vi "File Title Dialog.vi"() -> (1 "Accepted":bool, 2 "Additional Description out":string, 3 "File Title out":string="datafile_arduino")   [LabVIEW 2019]
panel:
  in  "Accept":bool
  in  "Additional Description":string
  in  "File Title":string="datafile_arduino"
  # "(no need to specify file extensions)"
  # "Numbers will be added if required to make the main filename unique."
  # "This will be written into the datafiles in the header, and can be left blank if desired. Commas are removed."
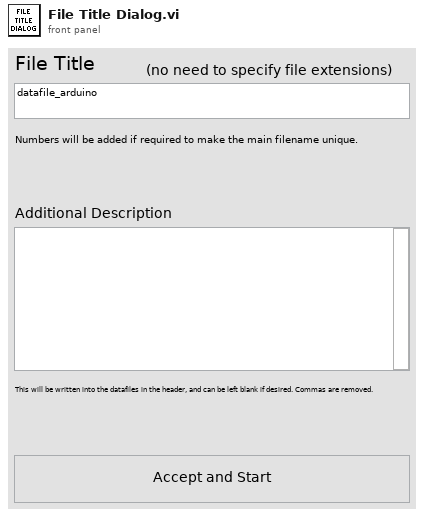
[diagram p1: front panel]
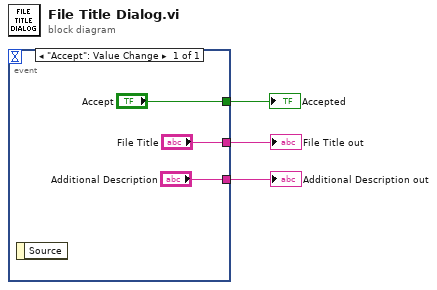
[diagram p0: block diagram]
diagram:
  n1 = event shown="[0] \"Accept\": Value Change" {
    selector: _ -> [_]
    dyn-events: _ -> [_]
    timeout: _ -> [_]
    tunnel: ["Accept"] -> w3
    tunnel: ["File Title"] -> w2
    tunnel: ["Additional Description"] -> w1
    event "Accept": Value Change {
      n2 = event-data() -> ()  [unwired: 1 in, 1 out]
    }
  }
  "Accepted" <- w3
  "Additional Description out" <- w1
  "File Title out" <- w2
